vi "BRig_dataCurrent_DAB_flipLR.vi"() -> (2 "output_DAB_flipLR":i32)   [LabVIEW 2014]
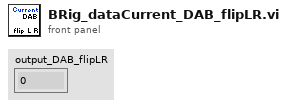
[diagram p1: front panel]
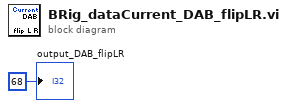
[diagram p0: block diagram]
diagram:
  "output_DAB_flipLR" <- 68 ("output_iBlock")
